vi "setUp.vi"(8 "error in (no error)":errorcluster, 11 "reference in":refnum<class "Test Osciloscope Module.lvclass">) -> (0 "error out":errorcluster, 3 "reference out":refnum<class "Test Osciloscope Module.lvclass">)   [LabVIEW 2020, in "Test Osciloscope Module.lvclass"]
doc: "setUp runs prior to the test method during test execution. Use this method to initialize any object data required by your tests."
uses:
  Test Osciloscope Module.lvclass
  C:/Program Files (x86)/National Instruments/LabVIEW 2020/vi.lib/addons/_JKI Toolkits/VI Tester/TestCase.llb/TestCase.lvclass
  Test Osciloscope Module.lvclass/Test Osciloscope Module.ctl
  <vilib>/addons/_JKI Toolkits/VI Tester/TestCase.llb/TestCase.lvclass
  Libraries/Osciloscope/Osciloscope.lvlib
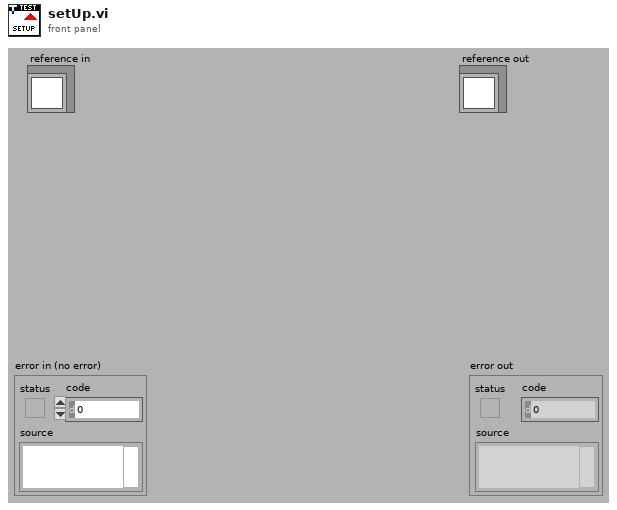
[diagram p1: front panel]
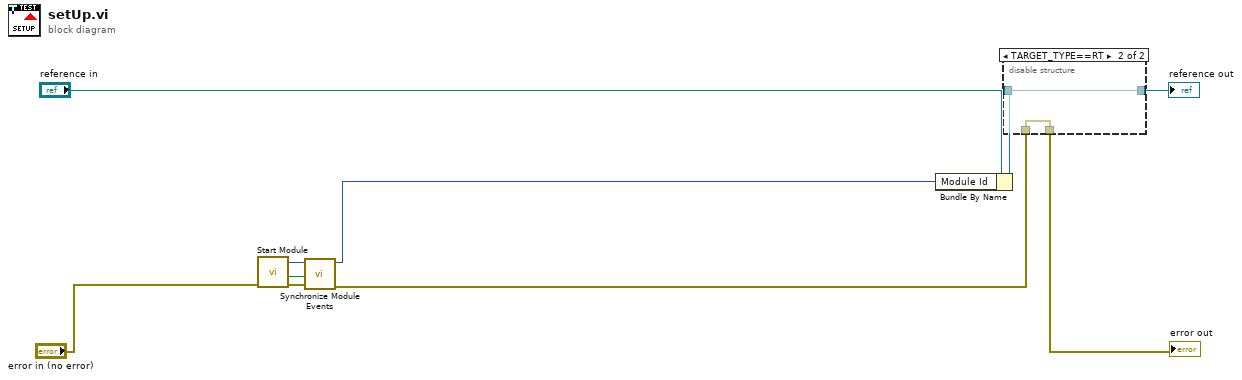
[diagram p0: block diagram]
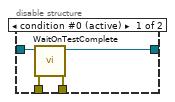
[diagram p2: hidden frame]
diagram:
  n1 = call "Start Module.vi"("error in"="error in (no error)") -> ("error out"=w5:errorcluster, "Wait for Event Sync?"=w2:bool, "Module ID"=w3:i32)  [unwired: 7 in, 1 out]
  n2 = call "Synchronize Module Events.vi"("error in"=w5, "Wait for Event Sync?"=w2, "Module ID in"=w3) -> ("error out"=w4:errorcluster, "Module ID out"=w1:i32)  [unwired: 7 in]
  n3 = Bundle By Name(cluster="reference in", "Module Id"=w1) -> (w7:refnum<class "Test Osciloscope Module.lvclass">)
  n4 = disable-structure shown="TARGET_TYPE==RT" {
    disable-tunnel: w4 -> [w14 w15]
    disable-tunnel: [w13 w15] -> w10
    disable-tunnel: [w12 w16] -> w8
    disable-tunnel: w7 -> [w11 w16]
    frame condition #0 (active) {
      n5 = call <vilib>:"WaitOnTestComplete.vi"("error in (no error)"=w14, "TestCase in"=w11) -> ("error out"=w13:errorcluster, "TestCase out"=w12:refnum<class "Test Osciloscope Module.lvclass">)  [unwired: 8 in]
    }
    frame condition #1 {
    }
  }
  "error out" <- w10
  "reference out" <- w8
